vi "Lian_Lab07_I.vi"() -> ()   [LabVIEW 2020]
uses:
  <vilib>/DAQmx/read.llb/DAQmx Read (Digital 1D Bool 1Chan 1Samp).vi
  <vilib>/DAQmx/create/channels.llb/DAQmx Create Channel (DI-Digital Input).vi
  <vilib>/DAQmx/miscellaneous.llb/DAQmx Fill In Error Info.vi
panel:
  out "?":bool[](array[boolean])
  in  "Line":tag="myDAQ1/port0/line0"
  in  "Loop Delay (ms)":u32
  in  "?":bool
  # "Part I."
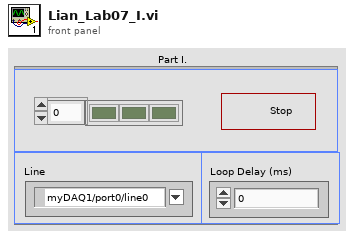
[diagram p1: front panel]
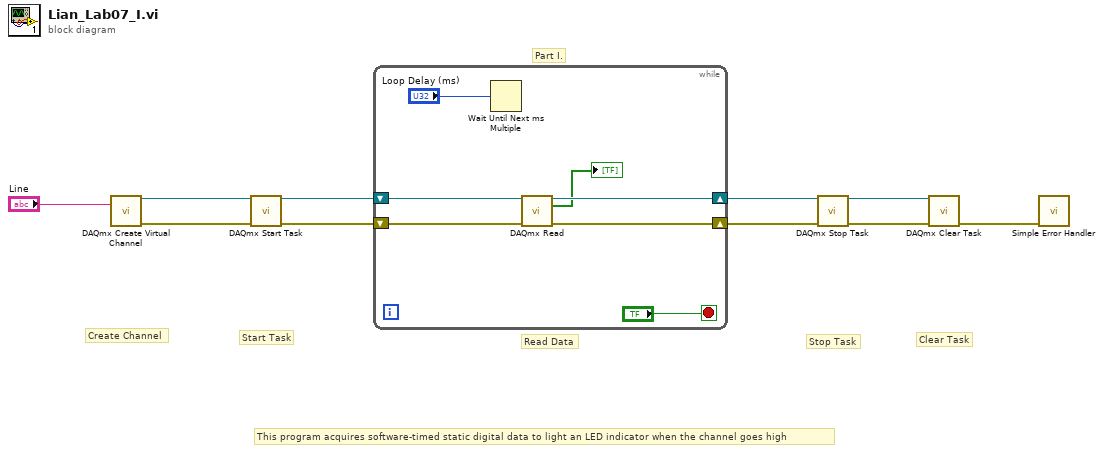
[diagram p0: block diagram]
diagram:
  # "This program acquires software-timed static digital data to light an LED indicator when the channel goes high"
  # "Read Data"
  # "Clear Task"
  # "Stop Task"
  # "Start Task"
  # "Create Channel"
  # "Part I."
  n1 = call-poly <vilib>:"DAQmx Create Virtual Channel.vi"("lines"="Line") -> ("task out"=w3:refnum<k21>, "error out"=w2:errorcluster)  [unwired: 13 in]
  n2 = call <vilib>:"DAQmx Start Task.vi"("task/channels in"=w3, "error in"=w2) -> ("task out"=w10:refnum<k21>, "error out"=w4:errorcluster)  [unwired: 12 in]
  n3 = while {
    shift-right: [w16] -> w9
    shift-left: w10 -> [w17]
    shift-right: [w14] -> w5
    shift-left: w4 -> [w15]
    stop <- "?" stop-if-true
    n4 = Wait Until Next ms Multiple(millisecond multiple="Loop Delay (ms)") -> ()  [unwired: 1 out]
    n5 = call-poly <vilib>:"DAQmx Read.vi"("task/channels in"=w17, "error in"=w15) -> ("task out"=w16:refnum<k21>, "data"=→"?":bool[], "error out"=w14:errorcluster)  [unwired: 11 in]
  }
  n6 = call <vilib>:"DAQmx Stop Task.vi"("task/channels in"=w9, "error in"=w5) -> ("task out"=w8:refnum<k21>, "error out"=w6:errorcluster)  [unwired: 12 in]
  n7 = call <vilib>:"DAQmx Clear Task.vi"("task in"=w8, "error in"=w6) -> ("error out"=w7:errorcluster)  [unwired: 13 in]
  n8 = call <vilib>:"Simple Error Handler.vi"("error in (no error)"=w7) -> ()  [unwired: 4 in, 5 out]
